vi "CRYInterpolate Post Data.vi"(9 "X value":dbl, 10 "Single Value":bool, 11 "Curve in":cluster{"x":dbl, "y":dbl}[](array[cluster])=[{"x"=10.0, "y"=2.0}, {"x"=20.0, "y"=6.0}]) -> (1 "Y value":dbl)   [LabVIEW 2013]
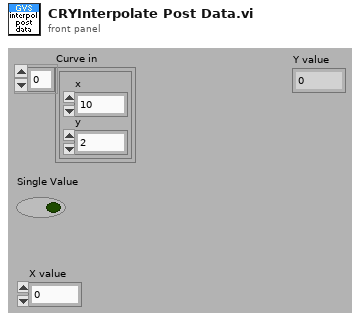
[diagram p1: front panel]
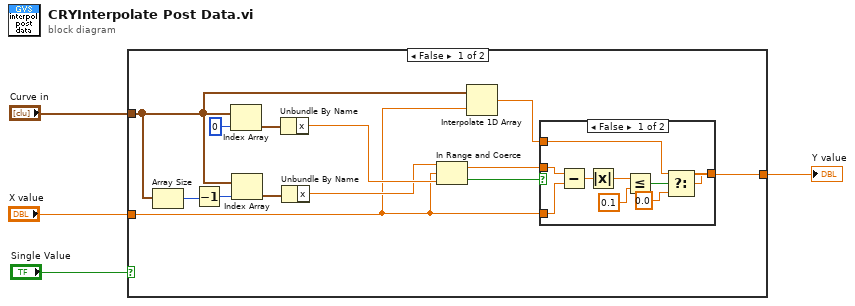
[diagram p0: block diagram]
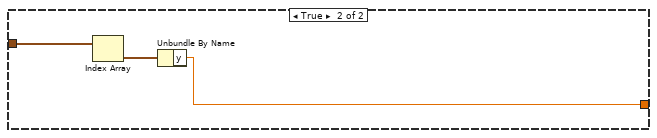
[diagram p3: hidden frame]
diagram:
  n1 = case shown="False" "Single Value" {
    tunnel: "X value" -> [w6 _]
    tunnel: "Curve in" -> [w12 w30]
    tunnel: [w7 w28] -> w2
    frame False {
      n2 = Array Size(array=w12) -> (size(s)=w15:i32)
      n3 = Decrement(x=w15) -> (x-1=w14:i32)
      n4 = Index Array(array=w12, index=0) -> (element=w17:cluster{"x":dbl, "y":dbl})
      n5 = Index Array(array=w12, index=w14) -> (element=w13:cluster{"x":dbl, "y":dbl})
      n6 = Unbundle By Name(w17) -> ("x"=w11:dbl)
      n7 = Unbundle By Name(w13) -> ("x"=w10:dbl)
      n8 = In Range and Coerce(upper limit=w10, x=w6, lower limit=w11) -> (coerced(x)=w5:dbl, In Range?=w8:bool)
      n9 = Interpolate 1D Array(1:w6, 2:w12) -> (0:w9:dbl)
      n10 = case shown="False" w8 {
        tunnel: w9 -> [w20 w27]
        tunnel: [w19 w27] -> w7
        tunnel: w6 -> [w25 _]
        tunnel: w5 -> [w26 _]
        frame False {
          n11 = Subtract(x=w26, y=w25) -> (x-y=w24:dbl)
          n12 = Absolute Value(x=w24) -> (abs(x)=w23:dbl)
          n13 = Less Or Equal?(x=w23, y=0.1) -> (x <= y?=w21:bool)
          n14 = Select(t=w20, s=w21, f=0.0) -> (s? t:f=w19:dbl)
        }
        frame True {
        }
      }
    }
    frame True {
      n15 = Index Array(array=w30) -> (element=w29:cluster{"x":dbl, "y":dbl})  [unwired: 1 in]
      n16 = Unbundle By Name(w29) -> ("y"=w28:dbl)
    }
  }
  "Y value" <- w2
